vi "PubVI_3.vi"(8 "error in (no error)":errorcluster, 11 "TestAgent in":refnum<class "TestAgent.lvclass">) -> (0 "error out":errorcluster, 3 "TestAgent out":refnum<class "TestAgent.lvclass">)   [LabVIEW 2009, in "TestAgent.lvlib" / "TestAgent.lvclass"]
uses:
  TestAgent.lvclass
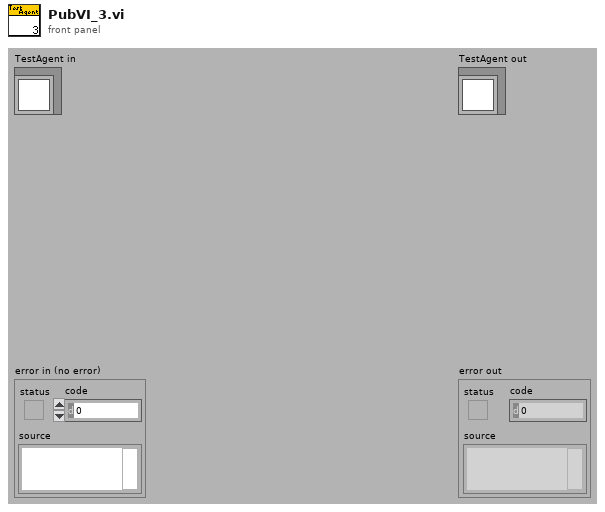
[diagram p1: front panel]
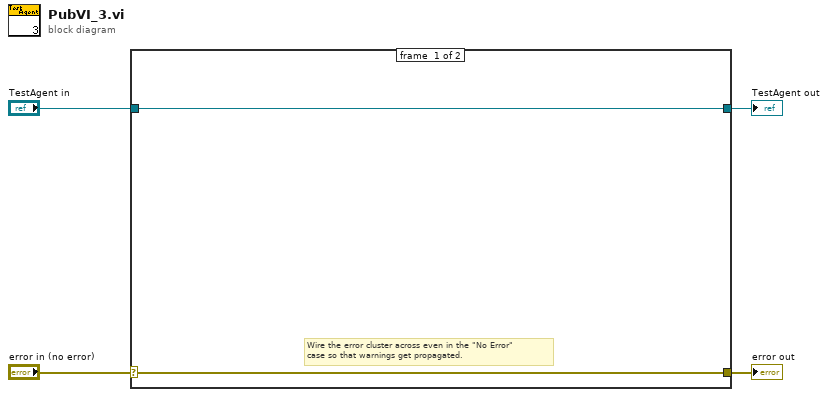
[diagram p0: block diagram]
diagram:
  n1 = case shown="No Error" "error in (no error)" {
    selector: "error in (no error)" -> [w5 w8]
    tunnel: [w5 w8] -> w3
    tunnel: [w6 w7] -> w1
    tunnel: "TestAgent in" -> [w6 w7]
    frame #0 {
      # "Wire the error cluster across even in the \"No Error\"\ncase so that warnings get propagated."
    }
    frame #1 {
    }
  }
  "error out" <- w3
  "TestAgent out" <- w1
